vi "Test_WriteValue_ReadValue_ValueReturned.vi"(8 "error in (no error)":errorcluster, 11 "TestCase in":refnum<class "TestValueReferenceTransport.lvclass">) -> (0 "error out":errorcluster, 3 "TestCase out":refnum<class "TestValueReferenceTransport.lvclass">)   [LabVIEW 2017, in "TestValueReferenceTransport.lvclass"]
uses:
  TestValueReferenceTransport.lvclass
  Source/Concrete/ValueReferenceTransport/ValueReferenceTransport.lvclass/ValueReferenceTransport.ctl
  Source/Concrete/ValueReferenceTransport/ValueReferenceTransport.lvclass
  C:/Git/composed-transport/Source/ITransport/ITransport.lvclass
  <vilib>/Utility/error.llb/Error Cluster From Error Code.vi
  Source/ITransport/ITransport.lvclass
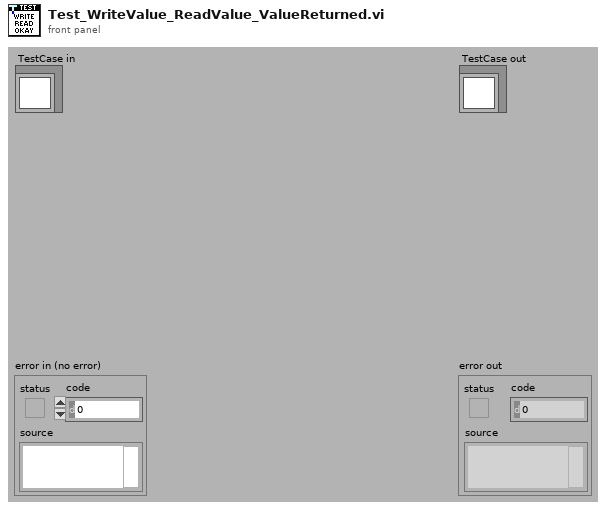
[diagram p1: front panel]
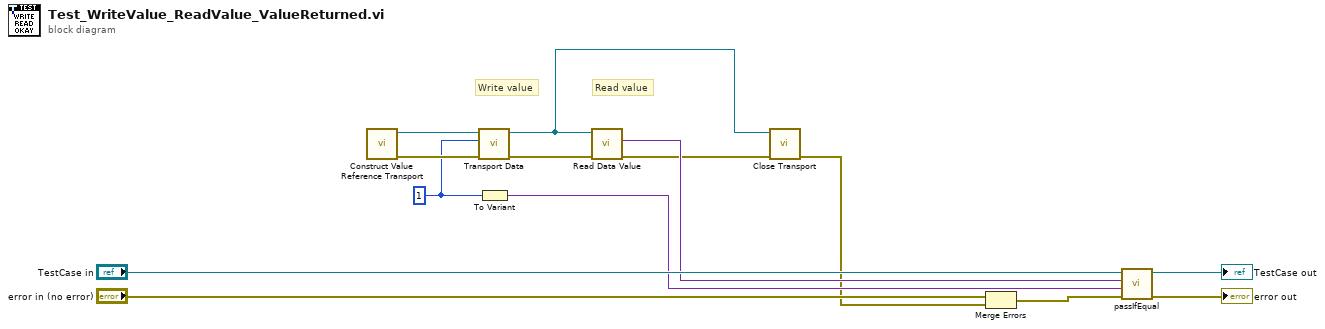
[diagram p0: block diagram]
diagram:
  w5 = 1
  # "Write value"
  # "Read value"
  n1 = call "Construct Value Reference Transport.vi"() -> ("error out"=w8:errorcluster, "ValueReferenceTransport"=w10:refnum<class "ValueReferenceTransport.lvclass">)  [unwired: 10 in]
  n2 = call "Transport Data.vi"("error in (no error)"=w8, "Value"=w5, "ITransport in"=w10) -> ("error out"=w7:errorcluster, "ITransport out"=w3:refnum<class "ValueReferenceTransport.lvclass">)  [unwired: 7 in]
  n3 = To Variant(anything=w5) -> (Variant=w4:variant)
  n4 = call "Read Data Value.vi"("error in (no error)"=w7, "ValueReferenceTransport In"=w3) -> ("error out"=w2:errorcluster, "Data"=w6:variant)  [unwired: 7 in, 1 out]
  n5 = call-dynamic "Close Transport.vi"("error in (no error)"=w2, "ValueReferenceTransport in"=w3) -> ("error out"=w1:errorcluster)  [unwired: 9 in]
  n6 = Merge Errors("error in (no error)", w1) -> (w9:errorcluster)
  n7 = call-dynamic "passIfEqual.vi"("error in (no error)"=w9, "y"=w4, "x"=w6, "TestCase in"="TestCase in") -> ("error out"=→"error out":errorcluster, "TestCase out"=→"TestCase out":refnum<class "TestValueReferenceTransport.lvclass">)  [unwired: 6 in]
